vi "Weather Simulator.vi"(11 "에러 입력(에러 없음)":errorcluster) -> (6 "웨이브폼 그래프":dynamicdata(graph), 15 "에러 출력":errorcluster)   [LabVIEW 2010]
doc: "이 VI는 5000 포인트로 50 kHz의 사인파의 온도와 전압을 생성합니다. 이 VI는 하드웨어를 이용할 수 없을 때 기상 관측기 프로젝트의 시뮬레이션으로서 사용됩니다."
uses:
  Instance           2 25Saved   Weather Simulator .vi
  Instance           1 25Saved   Weather Simulator .vi
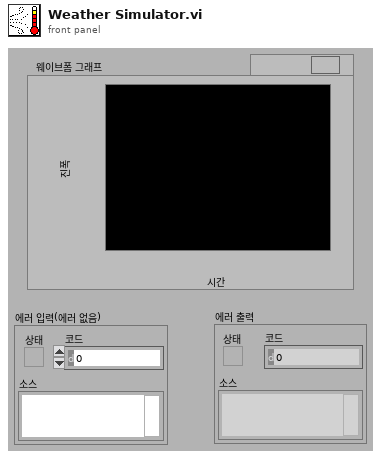
[diagram p1: front panel]
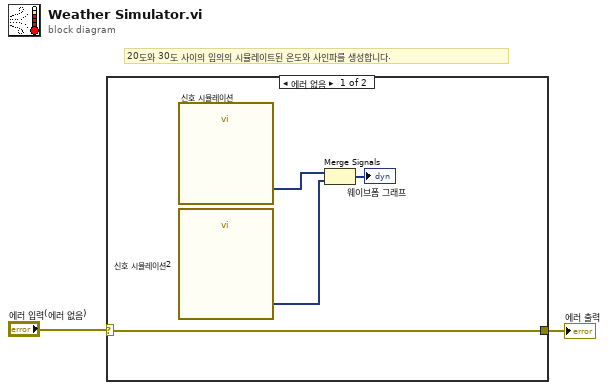
[diagram p0: block diagram]
diagram:
  # "20도와 30도 사이의 임의의 시뮬레이트된 온도와 사인파를 생성합니다."
  n1 = case shown="에러 없음" "에러 입력(에러 없음)" {
    selector: "에러 입력(에러 없음)" -> [w6 w7]
    tunnel: [w6 w7] -> w1
    frame No Error {
      n2 = call "신호 시뮬레이션"() -> ("온도"=w5:dynamicdata)  [unwired: 14 in, 1 out]
      n3 = call "신호 시뮬레이션2"() -> ("사인파"=w4:dynamicdata)  [unwired: 14 in, 1 out]
      n4 = Merge Signals(w5, w4) -> (→"웨이브폼 그래프":dynamicdata)
    }
    frame Error {
    }
  }
  "에러 출력" <- w1
